vi "Decrement.vi"(6 "Labels":map{string, string}(c390), 8 "error in (no error)":errorcluster, 10 "Step":dbl=1.0, 11 "Gauge Ref":refnum<data-value>) -> (0 "error out":errorcluster, 3 "Gauge Ref out":refnum<data-value>)   [LabVIEW 2020, in "Metrics.lvlib" / "Gauge.lvclass"]
doc: "Decrements the value of the gauge."
uses:
  Gauge.lvclass
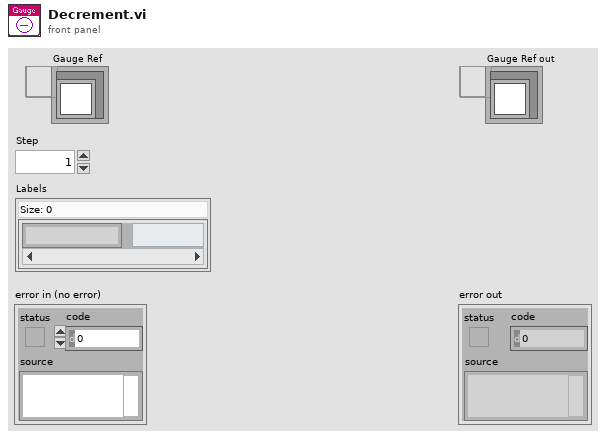
[diagram p1: front panel]
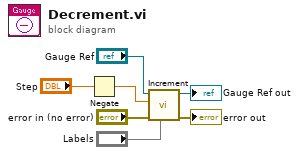
[diagram p0: block diagram]
diagram:
  n1 = Negate(x="Step") -> (-x=w4:dbl)
  n2 = call "Increment.vi"("Labels"="Labels", "error in (no error)"="error in (no error)", "Step"=w4, "Gauge Ref"="Gauge Ref") -> ("error out"=→"error out":errorcluster, "Gauge Ref out"=→"Gauge Ref out":refnum<data-value>)  [unwired: 6 in]
